vi "TestInkDictionary.vi"() -> ()   [LabVIEW 2022 SP3]
uses:
  Classes/TopLevel/Typedefs/processMode_parameters--cluster.ctl
  Controls/DLP_MaterialToHeadMapping--Cluster.ctl
  Classes/DLP2/DataTypes/DLP2_PrinterMaterialProperties.ctl
  Classes/TopLevel/Typedefs/InkIdleNodeConfigXML--Cluster.ctl
  Classes/TopLevel/Typedefs/InkProcessNodeConfigXML--Cluster.ctl
  <userlib>/_OpenG.lib/array/array.llb/Sort 1D Array (U8)__ogtk.vi
  <userlib>/_OpenG.lib/array/array.llb/Reorder 1D Array2 (String)__ogtk.vi
  <userlib>/_OpenG.lib/array/array.llb/Reorder 1D Array2 (Boolean)__ogtk.vi
  <userlib>/_OpenG.lib/array/array.llb/Reorder 1D Array2 (DBL)__ogtk.vi
  Classes/TopLevel/TopLevel.lvclass
panel:
  in  "PrinterInitialization.HIBEnable.#attributes":T1
  out "ProcessModeParams":T2
  in  "Recipe XML File Path":path
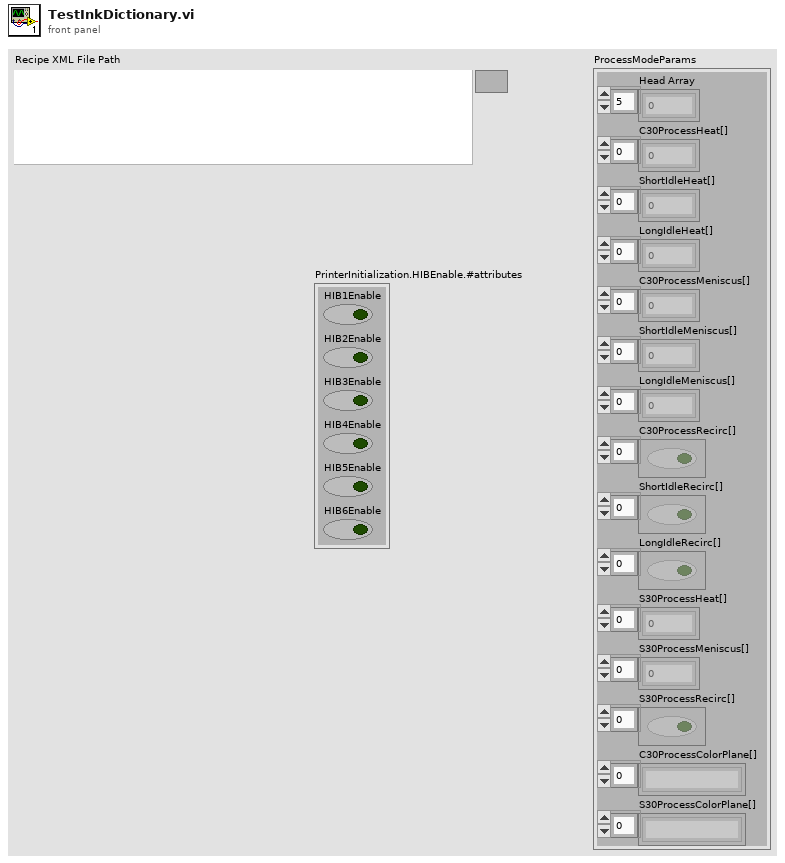
[diagram p1: front panel]
types:
  T1 = cluster{"HIB1Enable":bool, "HIB2Enable":bool, "HIB3Enable":bool, "HIB4Enable":bool, "HIB5Enable":bool, "HIB6Enable":bool}
  T2 = typedef "processMode_parameters--cluster.ctl" = cluster{"Head Array":u8[], "C30ProcessHeat[]":dbl[], "ShortIdleHeat[]":dbl[], "LongIdleHeat[]":dbl[], "C30ProcessMeniscus[]":dbl[], "ShortIdleMeniscus[]":dbl[], "LongIdleMeniscus[]":dbl[], "C30ProcessRecirc[]":bool[], "ShortIdleRecirc[]":bool[], "LongIdleRecirc[]":bool[], "S30ProcessHeat[]":dbl[], "S30ProcessMeniscus[]":dbl[], "S30ProcessRecirc[]":bool[], "C30ProcessColorPlane[]":string[], "S30ProcessColorPlane[]":string[]}
  T3 = typedef "DLPConfig_Initialization.ctl" = cluster{"PrinterInitialization":cluster{"Printer":cluster{"#attributes":cluster{"Name":string}}, "VacPumpSet":cluster{"#attributes":cluster{"VacPumpEnable":bool, "VacPumpSpeed":dbl}}, "HIBEnable":cluster{"#attributes":cluster{"HIB1Enable":bool, "HIB2Enable":bool, "HIB3Enable":bool, "HIB4Enable":bool, "HIB5Enable":bool, "HIB6Enable":bool}}, "PrinterCompensation":T4}, "HeadSet":cluster{"HeadProperties":T5[]}, "InkSet":cluster{"Ink":T7[]}, "Troubleshooting":cluster{"PMBLogging":cluster{"#attributes":cluster{"PMBMonitorDuringPrint":bool, "PMBMonitorDuringIdle":bool, "LogSwatheInputData":bool, "LogSwatheOutputData":bool, "LogPrintheadColourPlanes":bool, "LogPMBCommunication":bool, "LogSimulatedOutput":bool, "LogAllPMBCommunicationData":bool, "LogPMBSpace":bool, "ExtendedPMBSpaceLogging":bool, "LogPMBWriteSpeed":bool, "LogUsbRetries":bool}}, "HIBLogging":cluster{"#attributes":cluster{"HIBMonitoringDuringPrint":bool, "HIBMonitoringLog":bool}}}}
  T4 = typedef "DLP2_PrinterCompensationProperties.ctl" = cluster{"#attributes":cluster{"AppName":string, "PrintWeightMultiplier":dbl, "Rotation":bool, "Driver":string, "Server":string, "Database":string, "User":string, "Password":string}}
  T5 = typedef "DLP2_PrinterHeadProperties.ctl" = cluster{"#attributes":T6}
  T6 = typedef "DLPConfig)Init_HeadPropertyAttr--Cluster.ctl" = cluster{"HeadNumber":u8, "Material":string, "HeadLocalX":dbl, "HeadLocalY":dbl, "HeadRotationAngle":dbl, "VH2L_Hi":dbl, "VH2R_Hi":dbl, "VH1LA_Hi":dbl, "VH1LB_Hi":dbl, "VH1RA_Hi":dbl, "VH1RB_Hi":dbl, "VH2L_Lo":dbl, "VH2R_Lo":dbl, "VH1LA_Lo":dbl, "VH1LB_Lo":dbl, "VH1RA_Lo":dbl, "VH1RB_Lo":dbl}
  T7 = typedef "DLP2_PrinterMaterialProperties.ctl" = cluster{"#attributes":cluster{"InkType":string, "PrePrintPurge":bool, "PurgeTime":dbl, "PurgeCount":i32, "Density":dbl, "NumberofDrops":i32, "PrintWeight":dbl, "PrintheadPrime":bool}, "Idle":T8, "Process":T9}
  T8 = typedef "InkIdleNodeConfigXML--Cluster.ctl" = cluster{"ShortIdle":cluster{"#attributes":cluster{"Heat":dbl, "Meniscus":dbl, "Recirculation":bool}}, "LongIdle":cluster{"#attributes":cluster{"Heat":dbl, "Meniscus":dbl, "Recirculation":bool}}}
  T9 = typedef "InkProcessNodeConfigXML--Cluster.ctl" = cluster{"C30_Process":cluster{"#attributes":cluster{"Heat":dbl, "Meniscus":dbl, "Recirculation":bool, "ColorPlane":string}}, "S30_Process":cluster{"#attributes":cluster{"Heat":dbl, "Meniscus":dbl, "Recirculation":bool, "ColorPlane":string}}}
  T10 = typedef "DLP_MaterialToHeadMapping--Cluster.ctl" = cluster{"Head":u8, "Ink":T7}
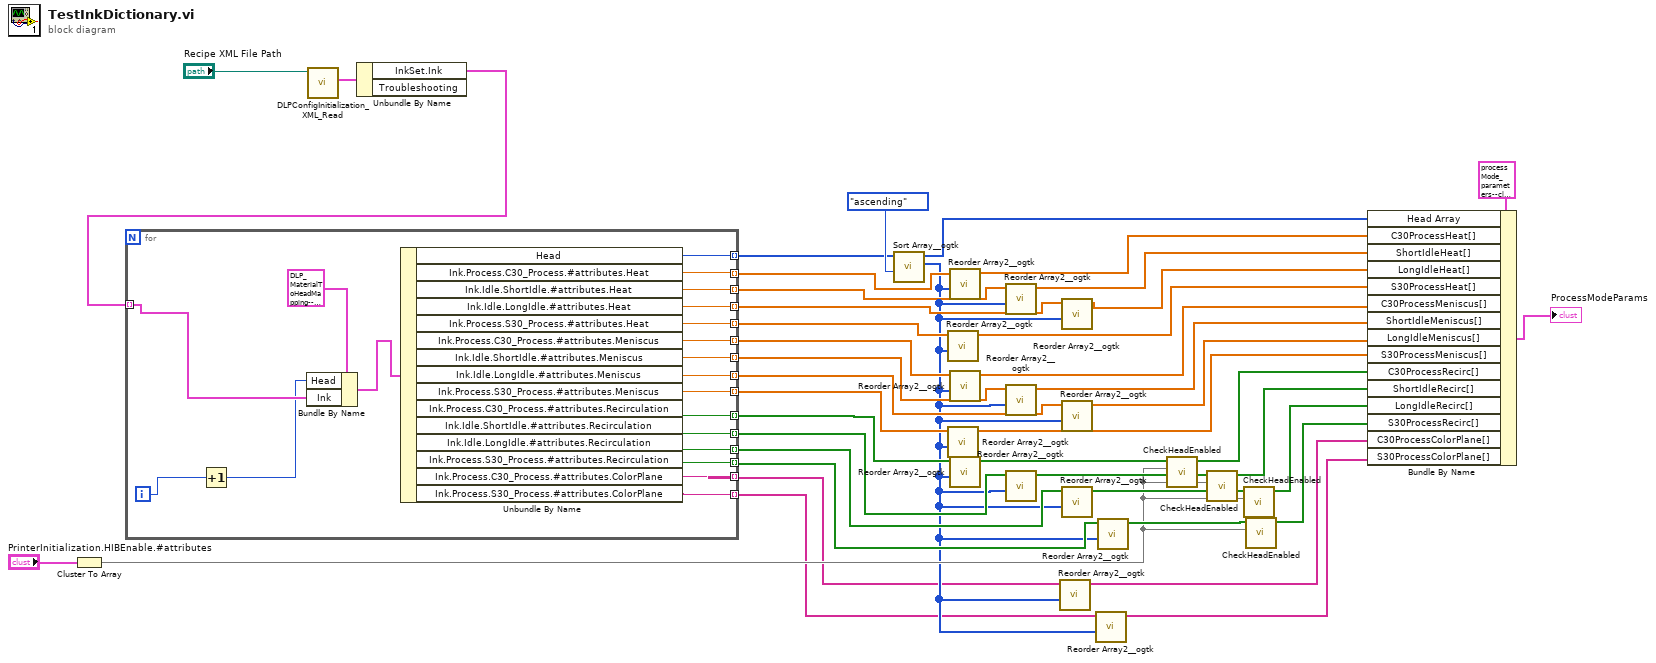
[diagram p0: block diagram]
diagram:
  n1 = Cluster To Array(cluster="PrinterInitialization.HIBEnable.#attributes") -> (array=w8:bool[])
  n2 = call "DLPConfigInitialization_XML_Read.vi"("Recipe XML File Path"="Recipe XML File Path") -> ("DLP"=w42:T3)  [unwired: 9 in, 1 out]
  n3 = Unbundle By Name(w42) -> ("InkSet.Ink"=w1:T7[])  [unwired: 1 out]
  n4 = for {
    tunnel: [w63] -> w31 mode=indexing
    tunnel: [w62] -> w33 mode=indexing
    tunnel: [w61] -> w34 mode=indexing
    tunnel: [w60] -> w35 mode=indexing
    tunnel: [w59] -> w30 mode=indexing
    tunnel: [w58] -> w29 mode=indexing
    tunnel: [w57] -> w28 mode=indexing
    tunnel: [w56] -> w24 mode=indexing
    tunnel: [w55] -> w23 mode=indexing
    tunnel: [w54] -> w22 mode=indexing
    tunnel: [w53] -> w14 mode=indexing
    tunnel: [w52] -> w13 mode=indexing
    tunnel: [w51] -> w10 mode=indexing
    tunnel: [w50] -> w5 mode=indexing
    tunnel: [w49] -> w4 mode=indexing
    tunnel: w1 -> [w46] mode=indexing
    i -> [w45]
    n5 = Increment(x=w45) -> (x+1=w44:i32)
    n6 = Bundle By Name(cluster=T10 {"Head"=0, "Ink"={"#attributes"={"InkType"="", "PrePrintPurge"=FALSE, "PurgeTime"=0.0, "PurgeCount"=0, "Density"=0.0, "NumberofDrops"=0, "PrintWeight"=0.0, "PrintheadPrime"=FALSE}, "Idle"={"ShortIdle"={"#attributes"={"Heat"=0.0, "Meniscus"=0.0, "Recirculation"=FALSE}}, "LongIdle"={"#attributes"={"Heat"=0.0, "Meniscus"=0.0, "Recirculation"=FALSE}}}, "Process"={"C30_Process"={"#attributes"={"Heat"=0.0, "Meniscus"=0.0, "Recirculation"=FALSE, "ColorPlane"=""}}, "S30_Process"={"#attributes"={"Heat"=0.0, "Meniscus"=0.0, "Recirculation"=FALSE, "ColorPlane"=""}}}}}, "Head"=w44, "Ink"=w46) -> (w47:T10)
    n7 = Unbundle By Name(w47) -> ("Head"=w63:u8, "Ink.Process.C30_Process.#attributes.Heat"=w62:dbl, "Ink.Idle.ShortIdle.#attributes.Heat"=w61:dbl, "Ink.Idle.LongIdle.#attributes.Heat"=w60:dbl, "Ink.Process.S30_Process.#attributes.Heat"=w53:dbl, "Ink.Process.C30_Process.#attributes.Meniscus"=w59:dbl, "Ink.Idle.ShortIdle.#attributes.Meniscus"=w58:dbl, "Ink.Idle.LongIdle.#attributes.Meniscus"=w57:dbl, "Ink.Process.S30_Process.#attributes.Meniscus"=w52:dbl, "Ink.Process.C30_Process.#attributes.Recirculation"=w56:bool, "Ink.Idle.ShortIdle.#attributes.Recirculation"=w55:bool, "Ink.Idle.LongIdle.#attributes.Recirculation"=w54:bool, "Ink.Process.S30_Process.#attributes.Recirculation"=w51:bool, "Ink.Process.C30_Process.#attributes.ColorPlane"=w50:string, "Ink.Process.S30_Process.#attributes.ColorPlane"=w49:string)
  }
  n8 = call-poly <userlib>:"Sort Array__ogtk.vi"("Order"=enum16{"ascending", "descending"}."ascending", "Array in"=w31) -> ("Sorted Pointers"=w6:i32[], "Sorted Array out"=w37:u8[])  [unwired: 8 in]
  n9 = call-poly <userlib>:"Reorder Array2__ogtk.vi"("indices"=w6, "array"=w14) -> ("reordered array"=w12:dbl[])  [unwired: 9 in]
  n10 = call-poly <userlib>:"Reorder Array2__ogtk.vi"("indices"=w6, "array"=w13) -> ("reordered array"=w11:dbl[])  [unwired: 9 in]
  n11 = call-poly <userlib>:"Reorder Array2__ogtk.vi"("indices"=w6, "array"=w33) -> ("reordered array"=w38:dbl[])  [unwired: 9 in]
  n12 = call-poly <userlib>:"Reorder Array2__ogtk.vi"("indices"=w6, "array"=w30) -> ("reordered array"=w27:dbl[])  [unwired: 9 in]
  n13 = call-poly <userlib>:"Reorder Array2__ogtk.vi"("indices"=w6, "array"=w24) -> ("reordered array"=w20:bool[])  [unwired: 9 in]
  n14 = call-poly <userlib>:"Reorder Array2__ogtk.vi"("indices"=w6, "array"=w34) -> ("reordered array"=w39:dbl[])  [unwired: 9 in]
  n15 = call-poly <userlib>:"Reorder Array2__ogtk.vi"("indices"=w6, "array"=w29) -> ("reordered array"=w26:dbl[])  [unwired: 9 in]
  n16 = call-poly <userlib>:"Reorder Array2__ogtk.vi"("indices"=w6, "array"=w23) -> ("reordered array"=w16:bool[])  [unwired: 9 in]
  n17 = call-poly <userlib>:"Reorder Array2__ogtk.vi"("indices"=w6, "array"=w5) -> ("reordered array"=w3:string[])  [unwired: 9 in]
  n18 = call-poly <userlib>:"Reorder Array2__ogtk.vi"("indices"=w6, "array"=w35) -> ("reordered array"=w41:dbl[])  [unwired: 9 in]
  n19 = call-poly <userlib>:"Reorder Array2__ogtk.vi"("indices"=w6, "array"=w28) -> ("reordered array"=w25:dbl[])  [unwired: 9 in]
  n20 = call-poly <userlib>:"Reorder Array2__ogtk.vi"("indices"=w6, "array"=w22) -> ("reordered array"=w18:bool[])  [unwired: 9 in]
  n21 = call-poly <userlib>:"Reorder Array2__ogtk.vi"("indices"=w6, "array"=w4) -> ("reordered array"=w2:string[])  [unwired: 9 in]
  n22 = call-poly <userlib>:"Reorder Array2__ogtk.vi"("indices"=w6, "array"=w10) -> ("reordered array"=w9:bool[])  [unwired: 9 in]
  n23 = call "CheckHeadEnabled.vi"("PrinterInitialization.HIBEnable.#attributes"=w8, "reordered array"=w20) -> ("Array"=w19:bool[])  [unwired: 9 in]
  n24 = call "CheckHeadEnabled.vi"("PrinterInitialization.HIBEnable.#attributes"=w8, "reordered array"=w16) -> ("Array"=w15:bool[])  [unwired: 9 in]
  n25 = call "CheckHeadEnabled.vi"("PrinterInitialization.HIBEnable.#attributes"=w8, "reordered array"=w18) -> ("Array"=w17:bool[])  [unwired: 9 in]
  n26 = call "CheckHeadEnabled.vi"("PrinterInitialization.HIBEnable.#attributes"=w8, "reordered array"=w9) -> ("Array"=w7:bool[])  [unwired: 9 in]
  n27 = Bundle By Name(cluster=T2 {"Head Array"=[], "C30ProcessHeat[]"=[], "ShortIdleHeat[]"=[], "LongIdleHeat[]"=[], "C30ProcessMeniscus[]"=[], "ShortIdleMeniscus[]"=[], "LongIdleMeniscus[]"=[], "C30ProcessRecirc[]"=[], "ShortIdleRecirc[]"=[], "LongIdleRecirc[]"=[], "S30ProcessHeat[]"=[], "S30ProcessMeniscus[]"=[], "S30ProcessRecirc[]"=[], "C30ProcessColorPlane[]"=[], "S30ProcessColorPlane[]"=[]}, "Head Array"=w37, "C30ProcessHeat[]"=w38, "ShortIdleHeat[]"=w39, "LongIdleHeat[]"=w41, "S30ProcessHeat[]"=w12, "C30ProcessMeniscus[]"=w27, "ShortIdleMeniscus[]"=w26, "LongIdleMeniscus[]"=w25, "S30ProcessMeniscus[]"=w11, "C30ProcessRecirc[]"=w19, "ShortIdleRecirc[]"=w15, "LongIdleRecirc[]"=w17, "S30ProcessRecirc[]"=w7, "C30ProcessColorPlane[]"=w3, "S30ProcessColorPlane[]"=w2) -> (→"ProcessModeParams":T2)
